vi "odor config array to odor-descrip map (sub-vi).vi"(10 "odor config array":T3) -> (2 "odor channel to description map":T1)   [LabVIEW 2021]
uses:
  type-defs/odor description array (type def).ctl
  type-defs/odor info cluster (type def).ctl
  type-defs/odor selection (type def).ctl
  type-defs/odor color (type def).ctl
  type-defs/odor channel to string map (type def).ctl
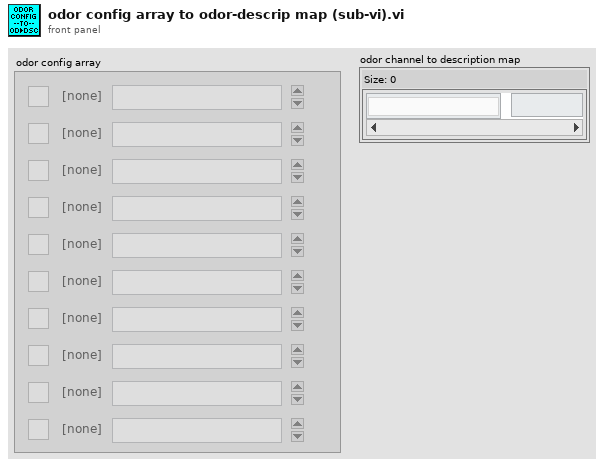
[diagram p1: front panel]
types:
  T1 = typedef "odor channel to string map (type def).ctl" = map{T2, string}
  T2 = typedef "odor selection (type def).ctl" = enum16{"[none]", "odor 1", "odor 2", "odor 3", "odor 4", "odor 5", "odor 6", "odor 7", "odor 8", "odor 9", "odor 10"}
  T3 = typedef "odor description array (type def).ctl" = T4[]
  T4 = typedef "odor info cluster (type def).ctl" = cluster{"odor channel":T2, "odor description":string, "odor color":T5, "odor channel active":bool}
  T5 = typedef "odor color (type def).ctl" = u16
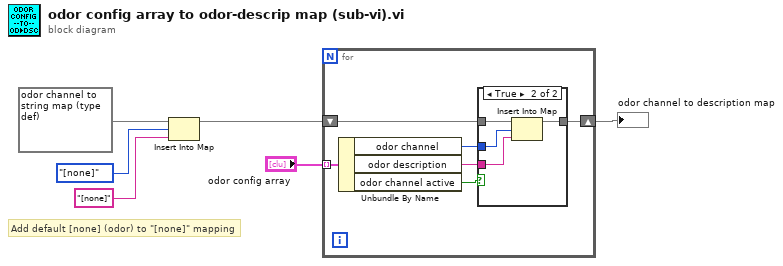
[diagram p0: block diagram]
diagram:
  # "Add default [none] (odor) to \"[none]\" mapping"
  n1 = Insert Into Map(map in=T1 {} ("Map"), key=odor_selection_(type_def)."[none]", value="[none]") -> (map out=w4:T1)  [unwired: 2 out]
  n2 = for {
    tunnel: "odor config array" -> [w12] mode=indexing
    shift-right: [w8] -> w6
    shift-left: w4 -> [w9]
    n3 = Unbundle By Name(w12) -> ("odor channel"=w11:T2, "odor description"=w10:string, "odor channel active"=w7:bool)
    n4 = case shown="True" w7 {
      tunnel: w11 -> [_ w17]
      tunnel: w10 -> [_ w16]
      tunnel: w9 -> [w13 w15]
      tunnel: [w13 w14] -> w8
      frame False {
      }
      frame True {
        n5 = Insert Into Map(map in=w15, key=w17, value=w16) -> (map out=w14:T1)  [unwired: 2 out]
      }
    }
  }
  "odor channel to description map" <- w6
